vi "Freq_FitnessCheck_Z.vi"(0 "alpha":dbl, 1 "beta":dbl[](array[numeric]), 2 "gamma":dbl, 3 "Omega":dbl[][](array[numeric]), 4 "q_input":dbl[](array[numeric])) -> (6 "fitness":dbl, 7 ">0":bool)   [LabVIEW 2015]
uses:
  <vilib>/Analysis/Matrix/Datatypes/RealMatrix.ctl
  <vilib>/Analysis/Matrix/Numeric/Conversions/Array To Matrix - RA.vi
  <vilib>/Analysis/Matrix/Numeric/Conversions/Array To Matrix - RA2.vi
  <vilib>/Analysis/Matrix/Numeric/Multiply/Multiply - RM,RM.vi
  <vilib>/Analysis/Matrix/NI_Matrix.lvlib
panel:
  out "q'*Omega*q":T1
  out "tmp1":dbl
  out "beta * q":T1
  out "tmp2":dbl
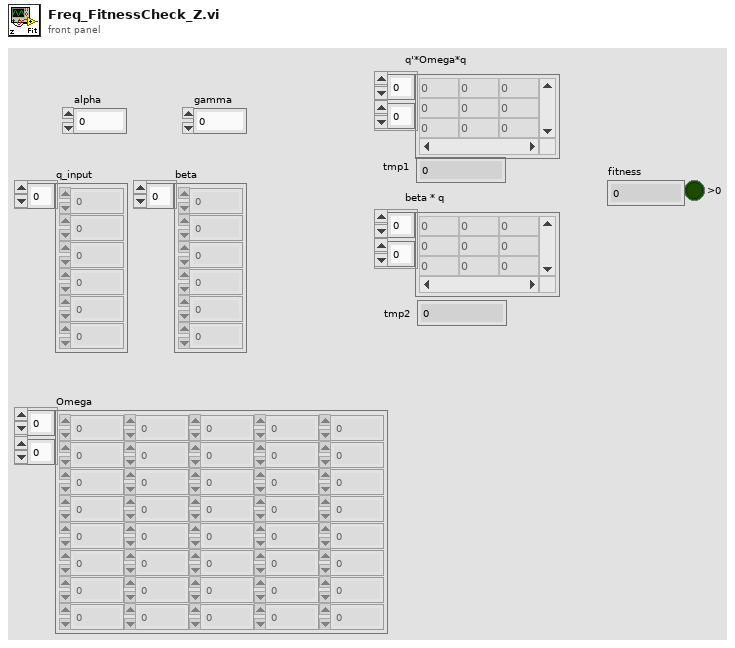
[diagram p1: front panel]
types:
  T1 = typedef "NI_Matrix.lvlib/RealMatrix.ctl" = dbl[][]
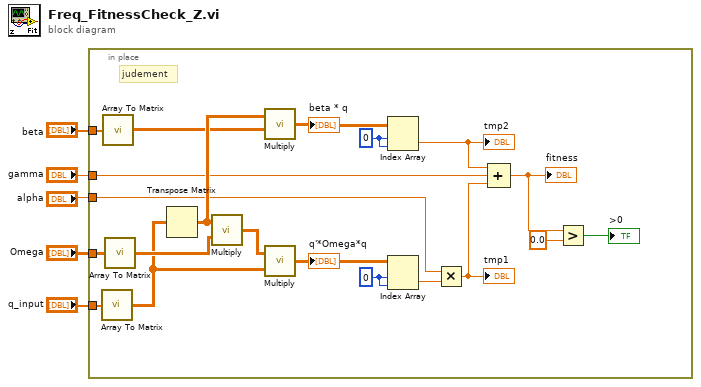
[diagram p0: block diagram]
diagram:
  n1 = in-place {
    in-place-border: "q_input" -> [w25]
    in-place-border: "gamma" -> [w14]
    in-place-border: "Omega" -> [w12]
    in-place-border: "alpha" -> [w11]
    in-place-border: "beta" -> [w10]
    w16 = 0 ("index (row)")
    w21 = 0 ("index (row)")
    # "judement"
    n2 = call-poly <vilib>:"Array To Matrix.vi"("Real 1D Array"=w25) -> ("Real Matrix (Column Vector)"=w19:T1)
    n3 = call-poly <vilib>:"Array To Matrix.vi"("Real 1D Array"=w10) -> ("Real Matrix (Column Vector)"=w17:T1)
    n4 = call-poly <vilib>:"Array To Matrix.vi"("Real 2D Array"=w12) -> ("Real Matrix"=w23:T1)
    n5 = Transpose Matrix(1:w19) -> (0:w18:T1)
    n6 = call-poly <vilib>:"Multiply.vi"("Real Matrix B"=w23, "Real Matrix A"=w18) -> ("A * B"=w24:T1)
    n7 = call-poly <vilib>:"Multiply.vi"("Real Matrix B"=w17, "Real Matrix A"=w18) -> ("A * B"=w9:T1)
    "beta * q" <- w9
    n8 = call-poly <vilib>:"Multiply.vi"("Real Matrix B"=w19, "Real Matrix A"=w24) -> ("A * B"=w22:T1)
    "q'*Omega*q" <- w22
    n9 = Index Array(array=w9, index (row)=w16, index (col)=w16) -> (element=w15:dbl)
    "tmp2" <- w15
    n10 = Index Array(array=w22, index (row)=w21, index (col)=w21) -> (element=w20:dbl)
    n11 = Multiply(x=w11, y=w20) -> (x*y=w13:dbl)
    "tmp1" <- w13
    n12 = Compound Arithmetic op=ADD(w15, w14, w13) -> (w7:dbl)
    "fitness" <- w7
    n13 = Greater?(x=w7, y=0.0) -> (0:→">0":bool)
  }
